vi "onTestDiscovery.vi"(8 "error in (no error)":errorcluster, 11 "Test Runner.Project in":refnum<class "Test Runner.Project.lvclass">) -> (0 "error out":errorcluster, 2 "Tests VIs":path[](array[path]), 3 "Test Runner.Project out":refnum<class "Test Runner.Project.lvclass">)   [LabVIEW 2013, in "Caraya.lvlib" / "Test Runner.Project.lvclass"]
uses:
  Test Runner.Project.lvclass
  Test Runner.Project.lvclass/Test Runner.Project.ctl
  Test Runner/Test Runner.lvclass/Test Runner.ctl
  Test Runner/Test Runner.lvclass
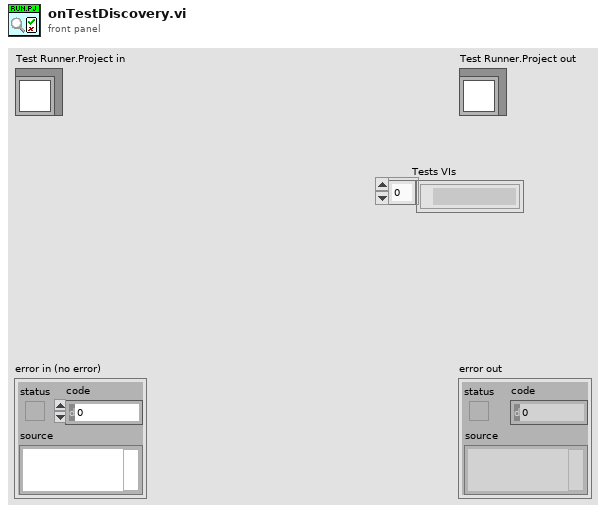
[diagram p1: front panel]
types:
  T1 = typedef "NI_FileType.lvlib/LVFileType.ctl" = enum32{"Invalid file", "Unknown type", "Instrument", "Control", "Polymorphic VI", "Project", "Library", "LVClass", "XControl", "XNode", "Shared library", ".NET assembly", "ActiveX interface", "CIN", "Run-time menu", "Palette menu", "Help file", "LLB", "XNode Edit Dependency", "Class Private Data Control", "Statechart", "MathScript .m file", "Ladder Diagram", "LVLibp", "XNode Build Dependency"}
  T2 = cluster{"path":path, "delimited name":string, "type":T1, "iState":u32, "iStyle":u16, "wStyle":u16, "buttons":u16, "viflags":u32, "viflags2":u32, "links":u32[]}[]
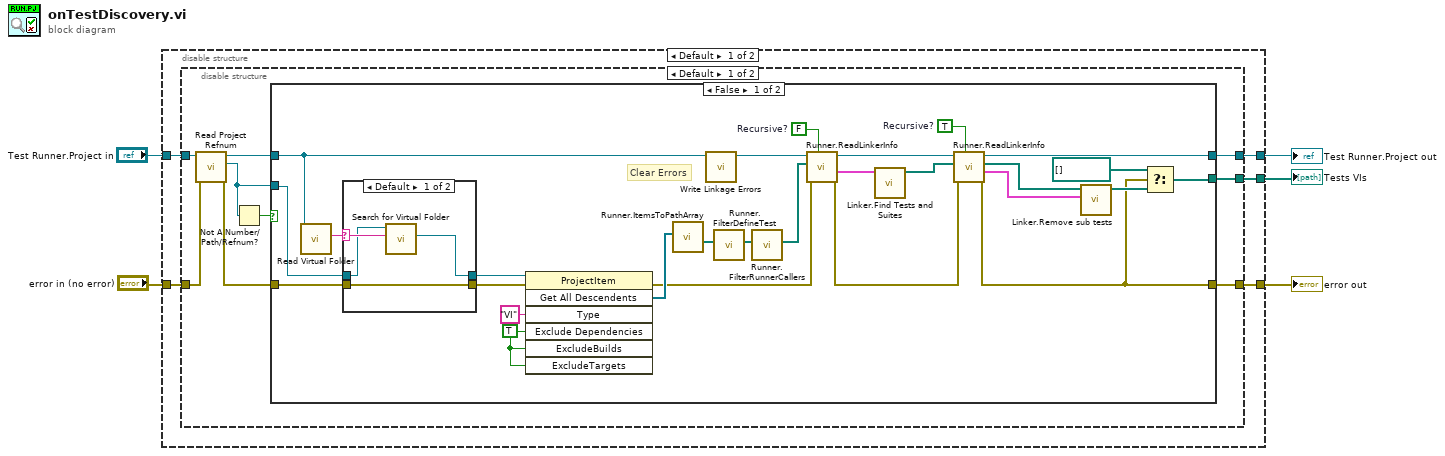
[diagram p0: block diagram]
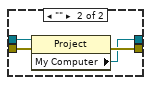
[diagram p2: hidden frame]
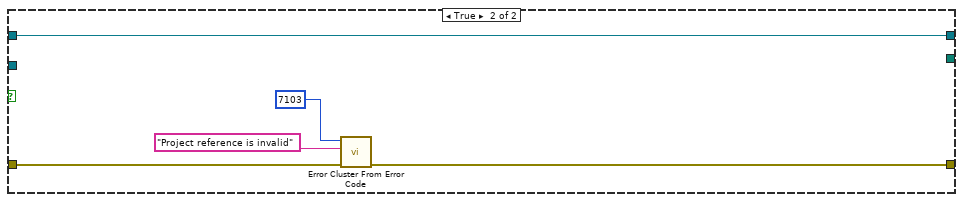
[diagram p3: hidden frame]
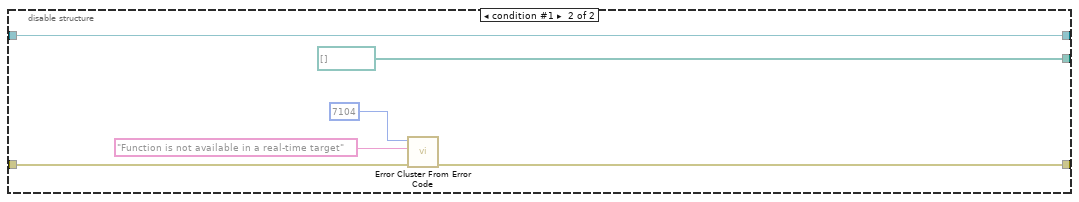
[diagram p4: hidden frame]
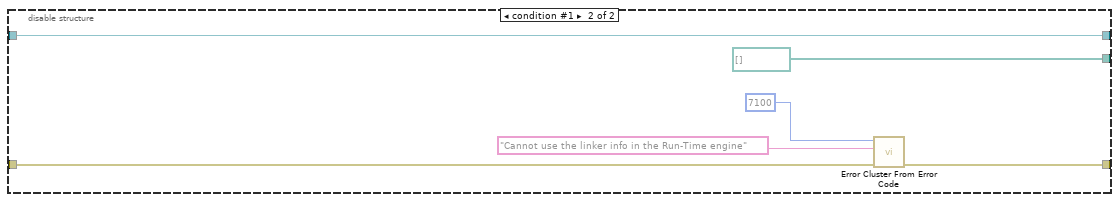
[diagram p5: hidden frame]
diagram:
  n1 = disable-structure shown="Default" {
    disable-tunnel: [w10 w69] -> w2
    disable-tunnel: "Test Runner.Project in" -> [w6 w68]
    disable-tunnel: [w9 w68] -> w3
    disable-tunnel: [w8 path[] [] ("Test VIs")] -> w1
    disable-tunnel: "error in (no error)" -> [w7 w66]
    frame condition #0 (active) {
      n2 = disable-structure shown="Default" {
        disable-tunnel: [w19 w61] -> w10
        disable-tunnel: [w18 w65] -> w9
        disable-tunnel: [w17 path[] [] ("Test VIs")] -> w8
        disable-tunnel: w7 -> [w15 w62]
        disable-tunnel: w6 -> [w13 w65]
        frame condition #0 (active) {
          n3 = call "Read Project Refnum.vi"("error in (no error)"=w15, "Test Runner.Project in"=w13) -> ("error out"=w14:errorcluster, "Project Refnum"=w11:refnum<vi>, "Test Runner.Project out"=w12:refnum<class "Test Runner.Project.lvclass">)  [unwired: 7 in]
          n4 = Not A Number/Path/Refnum?(number/path/refnum=w11) -> (NaN/Path/Refnum?=w16:bool)
          n5 = case shown="False" w16 {
            tunnel: [w26 w55] -> w19
            tunnel: [w46 _] -> w17
            tunnel: w11 -> [w39 _]
            tunnel: w12 -> [w31 w59]
            tunnel: [w27 w59] -> w18
            tunnel: w14 -> [w40 w56]
            frame False {
              w21 = FALSE  # Recursive?
              w20 = TRUE  # Recursive?
              w43 = TRUE ("ExcludeDependencies")
              # "Clear Errors"
              n6 = call "Read Virtual Folder.vi"("Test Runner.Project in"=w31) -> ("Virtual Folder"=w38:string)  [unwired: 9 in, 1 out]
              n7 = case shown="Default" w38 {
                selector: w38 -> [w50 _]
                tunnel: [w47 w54] -> w44
                tunnel: [w49 w51] -> w41
                tunnel: w40 -> [w47 w53]
                tunnel: w39 -> [w48 w52]
                frame Default {
                  n8 = call "Search for Virtual Folder.vi"("Virtual Folder"=w50, "Project Refnum"=w48) -> ("best match"=w49:refnum<vi>)  [unwired: 6 in, 3 out]
                }
                frame "" {
                  n9 = property class="Project"(reference=w52, error in=w53) -> (error out=w54:errorcluster, "My Computer"=w51:refnum<vi>)  [unwired: 1 out]
                }
              }
              n10 = invoke class="ProjectItem" method="Get All Descendents"(reference=w41, error in=w44, "Type"="VI", "Exclude Dependencies"=w43, "ExcludeBuilds"=w43, "ExcludeTargets"=w43) -> (error out=w32:errorcluster, "All Descendents"=w34:refnum<vi>[])  [unwired: 1 in, 5 out]
              n11 = call "Runner.ItemsToPathArray.vi"("Project Items"=w34) -> ("Paths"=w36:path[])  [unwired: 10 in]
              n12 = call "Write Linkage Errors.vi"("Test Runner in"=w31) -> ("Test Runner out"=w30:refnum<class "Test Runner.Project.lvclass">)  [unwired: 9 in, 1 out]
              n13 = call "Runner.FilterDefineTest.vi"("Paths"=w36) -> ("Filtered Paths"=w35:path[])  [unwired: 10 in]
              n14 = call "Runner.FilterRunnerCallers.vi"("Paths"=w35) -> ("Filtered Paths"=w33:path[])  [unwired: 10 in]
              n15 = call "Runner.ReadLinkerInfo.vi"("Recursive?"=w21, "error in (no error)"=w32, "VI Paths"=w33, "Test Runner in"=w30) -> ("error out"=w29:errorcluster, "Linker:Read Info From File"=w25:T2, "Test Runner out"=w28:refnum<class "Test Runner.Project.lvclass">)  [unwired: 4 in, 1 out]
              n16 = call "Linker.Find Tests and Suites.vi"("Linker:Read Info From File"=w25) -> ("All VIs defining a test (excluding those defining a suite)"=w23:path[])  [unwired: 8 in, 2 out]
              n17 = call "Runner.ReadLinkerInfo.vi"("Recursive?"=w20, "error in (no error)"=w29, "VI Paths"=w23, "Test Runner in"=w28) -> ("error out"=w26:errorcluster, "Linker:Read Info From File"=w24:T2, "VI Paths (dup)"=w22:path[], "Test Runner out"=w27:refnum<class "Test Runner.Project.lvclass">)  [unwired: 4 in]
              n18 = call "Linker.Remove sub tests.vi"("Linker.Read Info From File"=w24, "Tests"=w22) -> ("Array"=w37:path[])  [unwired: 9 in]
              n19 = Select(t=path[] [], s=w26, f=w37) -> (s? t:f=w46:path[])
            }
            frame True {
              n20 = call <vilib>:"Error Cluster From Error Code.vi"("error in (no error)"=w56, "error message (\"\")"="Project reference is invalid" ("error message (\"\")"), "error code (0)"=7103) -> ("error out"=w55:errorcluster)  [unwired: 6 in]
            }
          }
        }
        frame condition #1 {
          n21 = call <vilib>:"Error Cluster From Error Code.vi"("error in (no error)"=w62, "error message (\"\")"="Function is not available in a real-time target" ("error message (\"\")"), "error code (0)"=7104) -> ("error out"=w61:errorcluster)  [unwired: 6 in]
        }
      }
    }
    frame condition #1 {
      n22 = call <vilib>:"Error Cluster From Error Code.vi"("error in (no error)"=w66, "error message (\"\")"="Cannot use the linker info in the Run-Time engine" ("error message (\"\")"), "error code (0)"=7100) -> ("error out"=w69:errorcluster)  [unwired: 6 in]
    }
  }
  "error out" <- w2
  "Test Runner.Project out" <- w3
  "Tests VIs" <- w1
